vi "Table Index Up.vi"(7 "Table Index IN":i32, 8 "error in (no error)":errorcluster, 9 "UI Controls Refnum":T3, 10 "Image cluster":T1, 11 "Formatted Table Data":string[][](array[string])) -> (0 "error out":errorcluster, 2 "Table Index OUT":i32, 3 "Saved Image OUT":T2)   [LabVIEW 2012]
uses:
  Custom Control and Typedefs/UI Controls Refnum.ctl
  Custom Control and Typedefs/ChannelSelector_for_PosSave.ctl
  Custom Controls/PositionSaveMod.ctl
  Custom Control and Typedefs/Overlay Control.ctl
  <vilib>/vision/Image Controls.llb/IMAQ Image.ctl
  Custom Control and Typedefs/ImageCluster.ctl
  CommonResource VIs/FormatTableStyle_Commands.ctl
  SubVIs/ImageIO_commands.ctl
panel:
  # "Red (Current Image)"
  # "Green (Saved Image)"
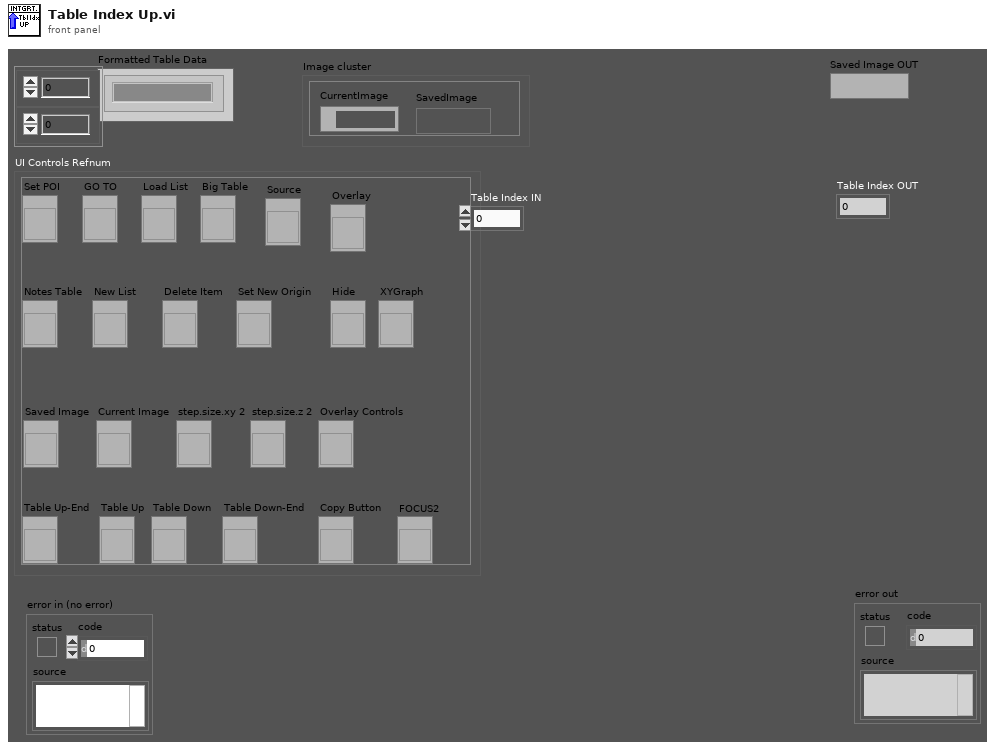
[diagram p1: front panel]
types:
  T1 = typedef "ImageCluster.ctl" = cluster{"CurrentImage":T2, "SavedImage":T2}
  T2 = typedef "IMAQ Image.ctl" = refnum<image>
  T3 = typedef "UI Controls Refnum.ctl" = cluster{"GO TO":refnum<vi>, "Load List":refnum<vi>, "Big Table":refnum<vi>, "Notes Table":refnum<vi>, "New List":refnum<vi>, "Delete Item":refnum<vi>, "Set New Origin":refnum<vi>, "Set POI":refnum<vi>, "Saved Image":refnum<vi>, "Current Image":refnum<vi>, "step.size.xy 2":refnum<vi>, "step.size.z 2":refnum<vi>, "Source":refnum<vi>, "Table Up-End":refnum<vi>, "Table Up":refnum<vi>, "Table Down":refnum<vi>, "Table Down-End":refnum<vi>, "Copy Button":refnum<vi>, "Hide":refnum<vi>, "Overlay Controls":refnum<vi>, "Overlay":refnum<vi>, "XYGraph":refnum<vi>, "FOCUS2":refnum<vi>}
  T4 = typedef "ImageIO_commands.ctl" = enum16{"ReadImage", "WriteImage"}
  T5 = typedef "FormatTableStyle_Commands.ctl" = enum16{"Colour Row", "Uncolour Row", "Bold Row", "Clear table", "UpdateVisibleRows"}
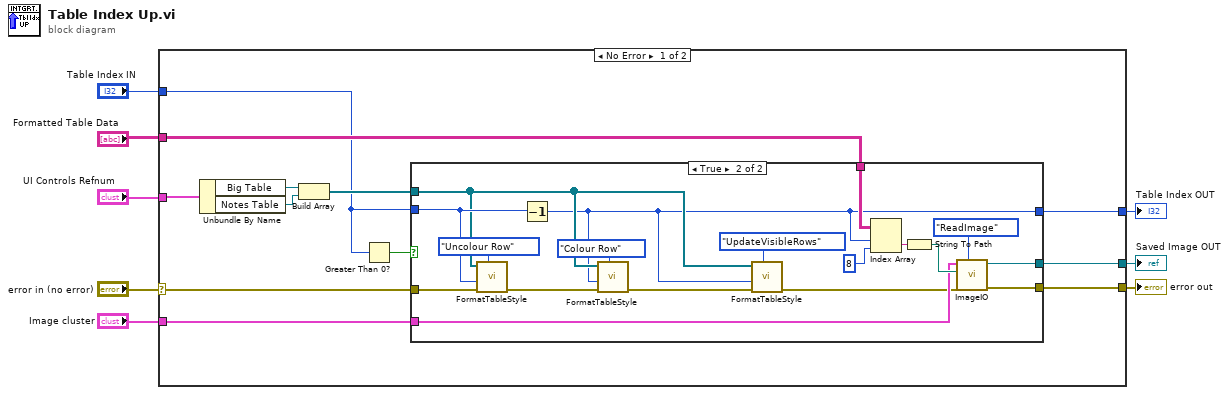
[diagram p0: block diagram]
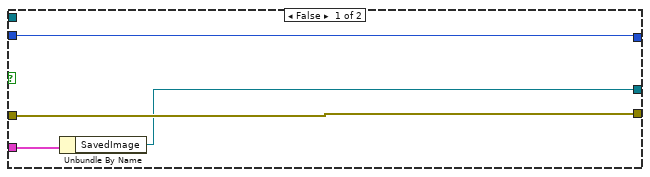
[diagram p2: hidden frame]
diagram:
  n1 = case shown="No Error" "error in (no error)" {
    selector: "error in (no error)" -> [w16 w43]
    tunnel: [w14 w43] -> w8
    tunnel: "Formatted Table Data" -> [w17 _]
    tunnel: "UI Controls Refnum" -> [w15 _]
    tunnel: [w13 _] -> w4
    tunnel: "Image cluster" -> [w12 _]
    tunnel: "Table Index IN" -> [w9 _]
    tunnel: [w11 _] -> w1
    frame No Error {
      n2 = Unbundle By Name(w15) -> ("Big Table"=w20:refnum<vi>, "Notes Table"=w19:refnum<vi>)
      n3 = Build Array(w20, w19) -> (w18:refnum<vi>[])
      n4 = Greater Than 0?(x=w9) -> (x > 0?=w10:bool)
      n5 = case shown="True" w10 {
        tunnel: w9 -> [w24 w42]
        tunnel: [w24 w33] -> w11
        tunnel: w18 -> [_ w35]
        tunnel: w16 -> [w23 w41]
        tunnel: [w23 w26] -> w14
        tunnel: w12 -> [w22 w28]
        tunnel: w17 -> [_ w34]
        tunnel: [w21 w25] -> w13
        frame False {
          n6 = Unbundle By Name(w22) -> ("SavedImage"=w21:T2)
        }
        frame True {
          n7 = call "FormatTableStyle.vi"("Format Command"=FormatTableStyle_Commands."Uncolour Row", "Error In"=w41, "Row Index"=w42, "Table reference Array"=w35) -> ("Error Out"=w40:errorcluster)  [unwired: 7 in]
          n8 = Decrement(x=w42) -> (x-1=w33:i32)
          n9 = call "FormatTableStyle.vi"("Format Command"=FormatTableStyle_Commands."Colour Row", "Error In"=w40, "Row Index"=w33, "Table reference Array"=w35) -> ("Error Out"=w36:errorcluster)  [unwired: 7 in]
          n10 = call "FormatTableStyle.vi"("Format Command"=FormatTableStyle_Commands."UpdateVisibleRows", "Error In"=w36, "Row Index"=w33, "Table reference Array"=w35) -> ("Error Out"=w27:errorcluster)  [unwired: 7 in]
          n11 = Index Array(array=w34, index (row)=w33, index (col)=8 ("disabled index (col)")) -> (element=w31:string)
          n12 = String To Path(string=w31) -> (path=w29:path)
          n13 = call "ImageIO.vi"("Pos_ImageIO_commands"=ImageIO_commands."ReadImage", "Error In"=w27, "Image File Path"=w29, "ImageCluster IN"=w28) -> ("Error Out"=w26:errorcluster, "Saved Image OUT"=w25:T2)  [unwired: 5 in, 1 out]
        }
      }
    }
    frame Error {
    }
  }
  "error out" <- w8
  "Saved Image OUT" <- w4
  "Table Index OUT" <- w1
